vi "SParam Fetch Result.vi"(8 "error in":errorcluster, 11 "S-Par Reference In":T1) -> (0 "error out":errorcluster, 1 "S-Param Magnitude":dbl[][](array[numeric]), 2 "S-Param Phase":dbl[][](array[numeric]), 3 "S-Par Reference Out":T1)   [LabVIEW 2023]
uses:
  <vilib>/niSPML/Typedefs/Session Handle.ctl
  <vilib>/niSPML/S-Par Reference.lvclass
  27770785-d40e-46c5-aceb-84cc9a890d04.vi
  <vilib>/niSPML/Fetch S-Parameters (All Complex).vi
  <vilib>/niSPML/S-Parameter Measurements.lvlib
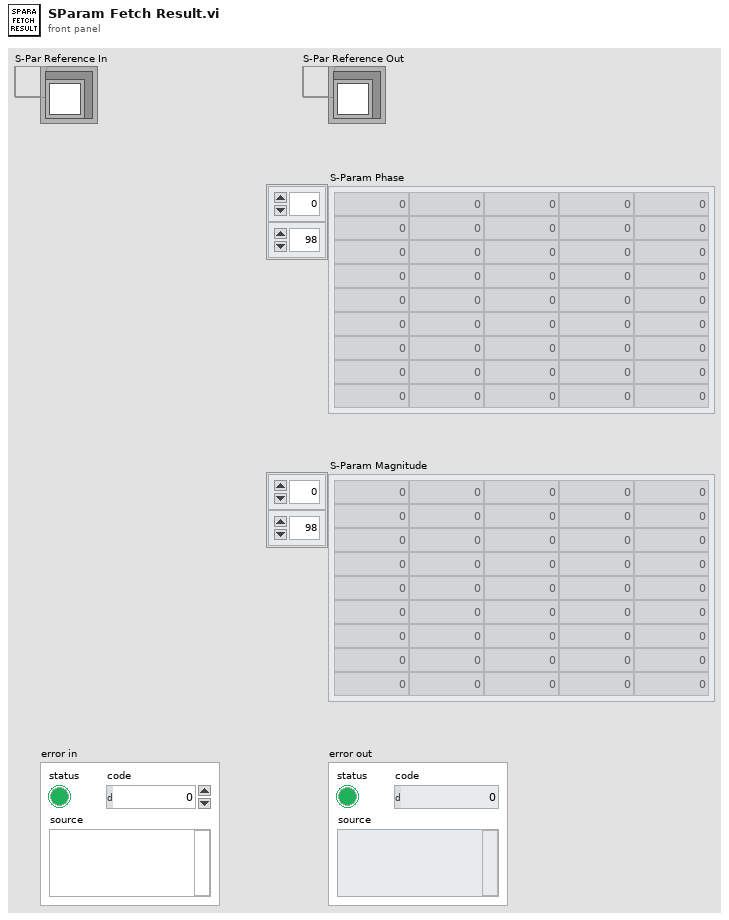
[diagram p1: front panel]
types:
  T1 = typedef "S-Parameter Measurements.lvlib/S-Par Reference.lvclass/Session Handle.ctl" = refnum<data-value>
  T2 = typedef "S-Parameter Measurements.lvlib/2d Complex 128 Array.ctl" = cdb[][]
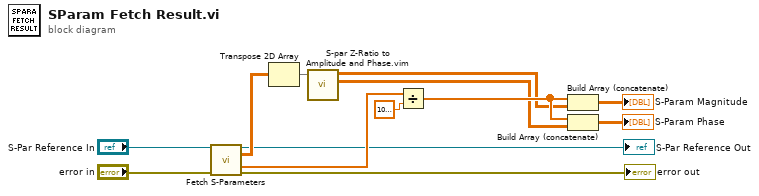
[diagram p0: block diagram]
diagram:
  n1 = call-poly <vilib>:"Fetch S-Parameters.vi"("S-Par Reference In"="S-Par Reference In", "error in"="error in") -> ("S-Par Reference Out"=→"S-Par Reference Out":T1, "S-Parameters"=w11:T2, "Frequency (Hz)"=w6:dbl[], "error out"=→"error out":errorcluster)  [unwired: 10 in]
  n2 = Transpose 2D Array(2D array=w11) -> (transposed array=w10:T2)
  n3 = call "S-par Z-Ratio to Amplitude and Phase.vim"("Z"=w10) -> ("Phase(degree)"=w3:dbl[][], "Amplitude(dB)"=w4:dbl[][])  [unwired: 8 in, 1 out]
  n4 = Divide(x=w6, y=1000000000.0 ("Frequency (Hz)")) -> (x/y=w5:dbl[])
  n5 = Build Array (concatenate)(w5, w4) -> (→"S-Param Magnitude":dbl[][])
  n6 = Build Array (concatenate)(w5, w3) -> (→"S-Param Phase":dbl[][])
